vi "Copy Files from Server.vi"(9 "Reg DAQ Rack Path":path, 10 "Cal Base Path":path, 11 "Server Support Path":path) -> (3 "Successful?":bool)   [LabVIEW 2019]
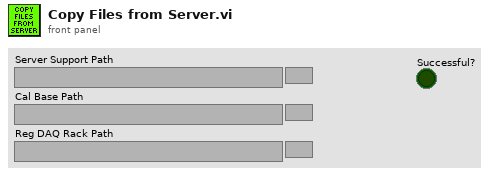
[diagram p1: front panel]
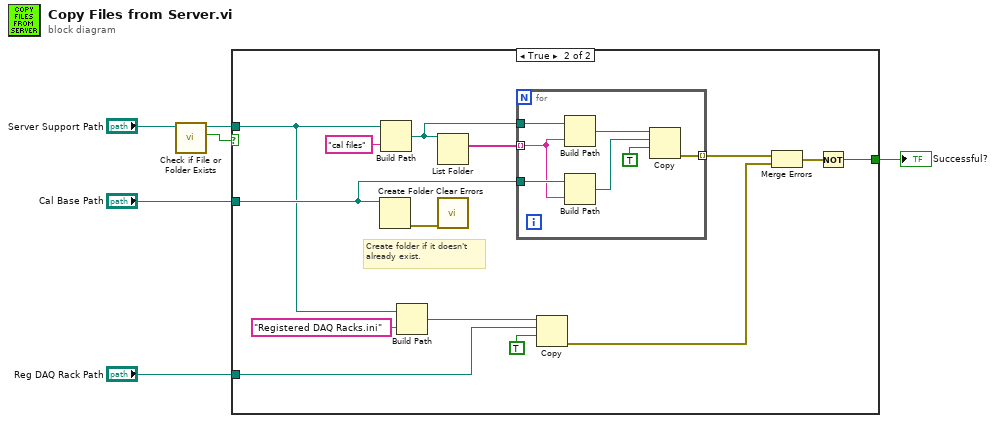
[diagram p0: block diagram]
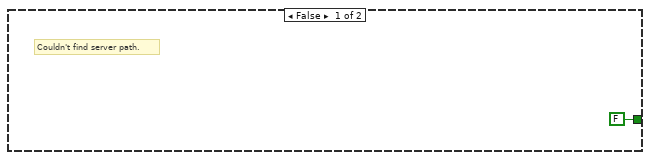
[diagram p2: hidden frame]
diagram:
  n1 = call <vilib>:"Check if File or Folder Exists.vi"("path"="Server Support Path") -> ("file or folder exists?"=w5:bool, "dup path"=w4:path)  [unwired: 8 in, 1 out]
  n2 = case shown="True" w5 {
    tunnel: w4 -> [_ w15]
    tunnel: "Cal Base Path" -> [_ w17]
    tunnel: "Reg DAQ Rack Path" -> [_ w12]
    tunnel: [FALSE w8] -> w1
    frame False {
      # "Couldn't find server path."
    }
    frame True {
      # "Create folder if it doesn't\nalready exist."
      n3 = Create Folder(path (use dialog)=w17) -> (error out=w20:errorcluster)  [unwired: 2 in, 2 out]
      n4 = Build Path(base path=w15, name or relative path="cal files") -> (appended path=w18:path)
      n5 = Build Path(base path=w15, name or relative path="Registered DAQ Racks.ini") -> (appended path=w13:path)
      n6 = List Folder(path=w18) -> (filenames=w19:string[])  [unwired: 3 in, 3 out]
      n7 = call <vilib>:"Clear Errors.vi"("error in (no error)"=w20) -> ()  [unwired: 5 in, 2 out]
      n8 = for {
        tunnel: w19 -> [w26] mode=indexing
        tunnel: w18 -> [w28]
        tunnel: w17 -> [w27]
        tunnel: [w22] -> w11 mode=indexing
        n9 = Build Path(base path=w28, name or relative path=w26) -> (appended path=w24:path)
        n10 = Build Path(base path=w27, name or relative path=w26) -> (appended path=w23:path)
        n11 = Copy(9:TRUE ("overwrite (F)"), 10:w23, 11:w24) -> (0:w22:errorcluster)  [unwired: 2 in, 2 out]
      }
      n12 = Copy(9:TRUE ("overwrite (F)"), 10:w12, 11:w13) -> (0:w10:errorcluster)  [unwired: 2 in, 2 out]
      n13 = Merge Errors(w11, w10) -> (w9:errorcluster)
      n14 = Not(x=w9) -> (.not. x?=w8:bool)
    }
  }
  "Successful?" <- w1
